vi "ListConfigurations.vi"(8 "Error In":errorcluster, 11 "reference in":refnum<class "AppConfigJSON.lvclass">) -> (0 "Error Out":errorcluster, 2 "Configurations":string[](array[string]), 3 "reference out":refnum<class "AppConfigJSON.lvclass">)   [LabVIEW 2021, in "AppConfigJSON.lvclass"]
uses:
  AppConfigJSON.lvclass
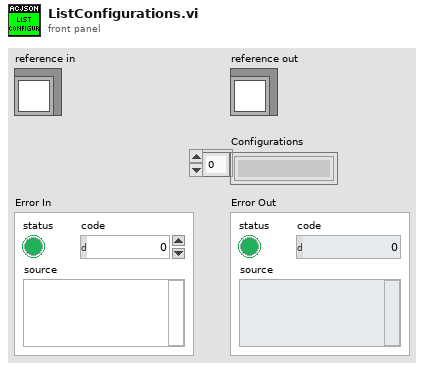
[diagram p1: front panel]
types:
  T1 = typedef "AppConfigJSON.lvclass/ObjectAttributes.ctl" = cluster{"Name":string, "ConfigFilePath":path, "Objects":T2[], "ApplicationBasePath":path}
  T2 = typedef "IApplicationConfiguration.lvclass/ObjectDataDetails.ctl" = cluster{"ObjectName":string, "ObjectType":string, "Interfaces":T3[]}
  T3 = typedef "IApplicationConfiguration.lvclass/ObjectData.ctl" = cluster{"Label":string, "ObjectName":string}
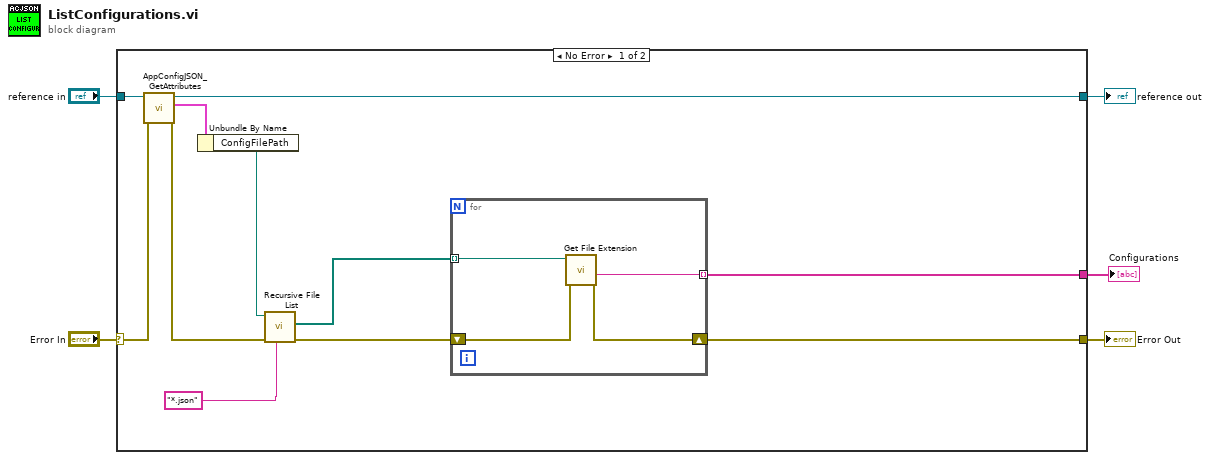
[diagram p0: block diagram]
diagram:
  n1 = case shown="No Error" "Error In" {
    selector: "Error In" -> [w15 w21]
    tunnel: [w7 w21] -> w4
    tunnel: [w12 w20] -> w2
    tunnel: "reference in" -> [w13 w20]
    tunnel: [w9 _] -> w1
    frame No Error {
      n2 = call "AppConfigJSON_GetAttributes.vi"("error in (no error)"=w15, "reference in"=w13) -> ("error out"=w8:errorcluster, "Data"=w14:T1, "reference out"=w12:refnum<class "AppConfigJSON.lvclass">)  [unwired: 6 in, 1 out]
      n3 = Unbundle By Name(w14) -> ("ConfigFilePath"=w11:path)
      n4 = call <vilib>:"Recursive File List.vi"("pattern"="*.json" ("string"), "error in (no error)"=w8, "Folder Path"=w11) -> ("All Files in Dir"=w10:path[])  [unwired: 4 in, 4 out]
      n5 = for {
        tunnel: w10 -> [w19] mode=indexing
        tunnel: [w18] -> w9 mode=indexing
        shift-right: [w16] -> w7
        shift-left: w8 -> [w17]
        n6 = call <vilib>:"Get File Extension.vi"("error in (no error)"=w17, "file"=w19) -> ("error out"=w16:errorcluster, "filename without extension"=w18:string)  [unwired: 5 in, 3 out]
      }
    }
    frame Error {
    }
  }
  "Error Out" <- w4
  "reference out" <- w2
  "Configurations" <- w1
